vi "custom_2_stimulus_setup.vi"(1 "input cluster":T1) -> (0 "output cluster":T2)   [LabVIEW 2010]
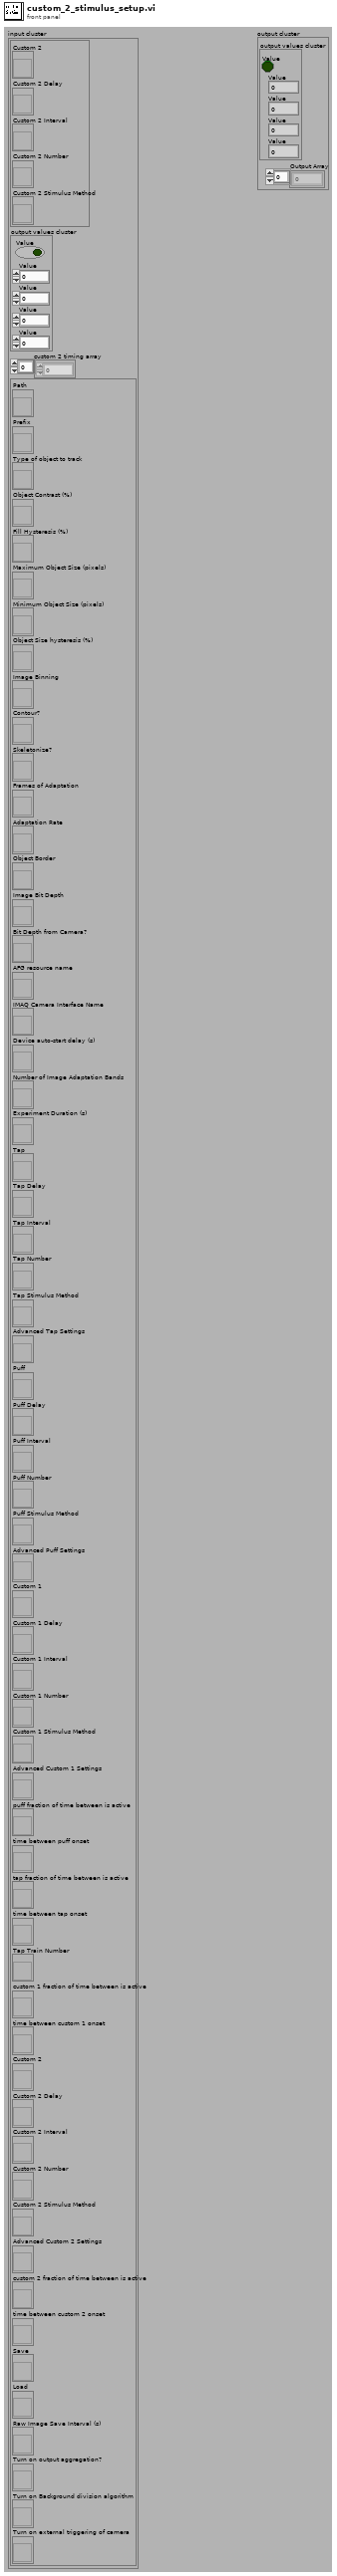
[diagram p1: front panel]
types:
  T1 = cluster{cluster{"Custom 2":refnum<vi>, "Custom 2 Delay":refnum<vi>, "Custom 2 Interval":refnum<vi>, "Custom 2 Number":refnum<vi>, "Custom 2 Stimulus Method":refnum<vi>}, "output values cluster":cluster{"Value":bool, "Value":dbl, "Value":dbl, "Value":dbl, "Value":u16}, "custom 2 timing array":dbl[], cluster{"Path":refnum<vi>, "Prefix":refnum<vi>, "Type of object to track":refnum<vi>, "Object Contrast (%)":refnum<vi>, "Fill Hysteresis (%)":refnum<vi>, "Maximum Object Size (pixels)":refnum<vi>, "Minimum Object Size (pixels)":refnum<vi>, "Object Size hysteresis (%)":refnum<vi>, "Image Binning":refnum<vi>, "Contour?":refnum<vi>, "Skeletonize?":refnum<vi>, "Frames of Adaptation":refnum<vi>, "Adaptation Rate":refnum<vi>, "Object Border":refnum<vi>, "Image Bit Depth":refnum<vi>, "Bit Depth from Camera?":refnum<vi>, "AFG resource name":refnum<vi>, "IMAQ Camera Interface Name":refnum<vi>, "Device auto-start delay (s)":refnum<vi>, "Number of Image Adaptation Bands":refnum<vi>, "Experiment Duration (s)":refnum<vi>, "Tap":refnum<vi>, "Tap Delay":refnum<vi>, "Tap Interval":refnum<vi>, "Tap Number":refnum<vi>, "Tap Stimulus Method":refnum<vi>, "Advanced Tap Settings":refnum<vi>, "Puff":refnum<vi>, "Puff Delay":refnum<vi>, "Puff Interval":refnum<vi>, "Puff Number":refnum<vi>, "Puff Stimulus Method":refnum<vi>, "Advanced Puff Settings":refnum<vi>, "Custom 1":refnum<vi>, "Custom 1 Delay":refnum<vi>, "Custom 1 Interval":refnum<vi>, "Custom 1 Number":refnum<vi>, "Custom 1 Stimulus Method":refnum<vi>, "Advanced Custom 1 Settings":refnum<vi>, "puff fraction of time between is active":refnum<vi>, "time between puff onset":refnum<vi>, "tap fraction of time between is active":refnum<vi>, "time between tap onset":refnum<vi>, "Tap Train Number":refnum<vi>, "custom 1 fraction of time between is active":refnum<vi>, "time between custom 1 onset":refnum<vi>, "Custom 2":refnum<vi>, "Custom 2 Delay":refnum<vi>, "Custom 2 Interval":refnum<vi>, "Custom 2 Number":refnum<vi>, "Custom 2 Stimulus Method":refnum<vi>, "Advanced Custom 2 Settings":refnum<vi>, "custom 2 fraction of time between is active":refnum<vi>, "time between custom 2 onset":refnum<vi>, "Save":refnum<vi>, "Load":refnum<vi>, "Raw Image Save Interval (s)":refnum<vi>, "Turn on output aggregation?":refnum<vi>, "Turn on Background division algorithm":refnum<vi>, "Turn on external triggering of camera":refnum<vi>}}
  T2 = cluster{"output values cluster":cluster{"Value":bool, "Value":dbl, "Value":dbl, "Value":dbl, "Value":u16}, "Output Array":dbl[]}
  T3 = cluster{"Custom 2":refnum<vi>, "Custom 2 Delay":refnum<vi>, "Custom 2 Interval":refnum<vi>, "Custom 2 Number":refnum<vi>, "Custom 2 Stimulus Method":refnum<vi>}
  T4 = cluster{"Value":bool, "Value":dbl, "Value":dbl, "Value":dbl, "Value":u16}
  T5 = cluster{"Path":refnum<vi>, "Prefix":refnum<vi>, "Type of object to track":refnum<vi>, "Object Contrast (%)":refnum<vi>, "Fill Hysteresis (%)":refnum<vi>, "Maximum Object Size (pixels)":refnum<vi>, "Minimum Object Size (pixels)":refnum<vi>, "Object Size hysteresis (%)":refnum<vi>, "Image Binning":refnum<vi>, "Contour?":refnum<vi>, "Skeletonize?":refnum<vi>, "Frames of Adaptation":refnum<vi>, "Adaptation Rate":refnum<vi>, "Object Border":refnum<vi>, "Image Bit Depth":refnum<vi>, "Bit Depth from Camera?":refnum<vi>, "AFG resource name":refnum<vi>, "IMAQ Camera Interface Name":refnum<vi>, "Device auto-start delay (s)":refnum<vi>, "Number of Image Adaptation Bands":refnum<vi>, "Experiment Duration (s)":refnum<vi>, "Tap":refnum<vi>, "Tap Delay":refnum<vi>, "Tap Interval":refnum<vi>, "Tap Number":refnum<vi>, "Tap Stimulus Method":refnum<vi>, "Advanced Tap Settings":refnum<vi>, "Puff":refnum<vi>, "Puff Delay":refnum<vi>, "Puff Interval":refnum<vi>, "Puff Number":refnum<vi>, "Puff Stimulus Method":refnum<vi>, "Advanced Puff Settings":refnum<vi>, "Custom 1":refnum<vi>, "Custom 1 Delay":refnum<vi>, "Custom 1 Interval":refnum<vi>, "Custom 1 Number":refnum<vi>, "Custom 1 Stimulus Method":refnum<vi>, "Advanced Custom 1 Settings":refnum<vi>, "puff fraction of time between is active":refnum<vi>, "time between puff onset":refnum<vi>, "tap fraction of time between is active":refnum<vi>, "time between tap onset":refnum<vi>, "Tap Train Number":refnum<vi>, "custom 1 fraction of time between is active":refnum<vi>, "time between custom 1 onset":refnum<vi>, "Custom 2":refnum<vi>, "Custom 2 Delay":refnum<vi>, "Custom 2 Interval":refnum<vi>, "Custom 2 Number":refnum<vi>, "Custom 2 Stimulus Method":refnum<vi>, "Advanced Custom 2 Settings":refnum<vi>, "custom 2 fraction of time between is active":refnum<vi>, "time between custom 2 onset":refnum<vi>, "Save":refnum<vi>, "Load":refnum<vi>, "Raw Image Save Interval (s)":refnum<vi>, "Turn on output aggregation?":refnum<vi>, "Turn on Background division algorithm":refnum<vi>, "Turn on external triggering of camera":refnum<vi>}
  T6 = cluster{"custom 2 fraction of time between is active":refnum<vi>, "time between custom 2 onset":refnum<vi>}
  T7 = cluster{"Custom":refnum<vi>, "Custom Delay":refnum<vi>, "Custom Interval":refnum<vi>, "Custom Number":refnum<vi>, "Custom Stimulus Method":refnum<vi>}
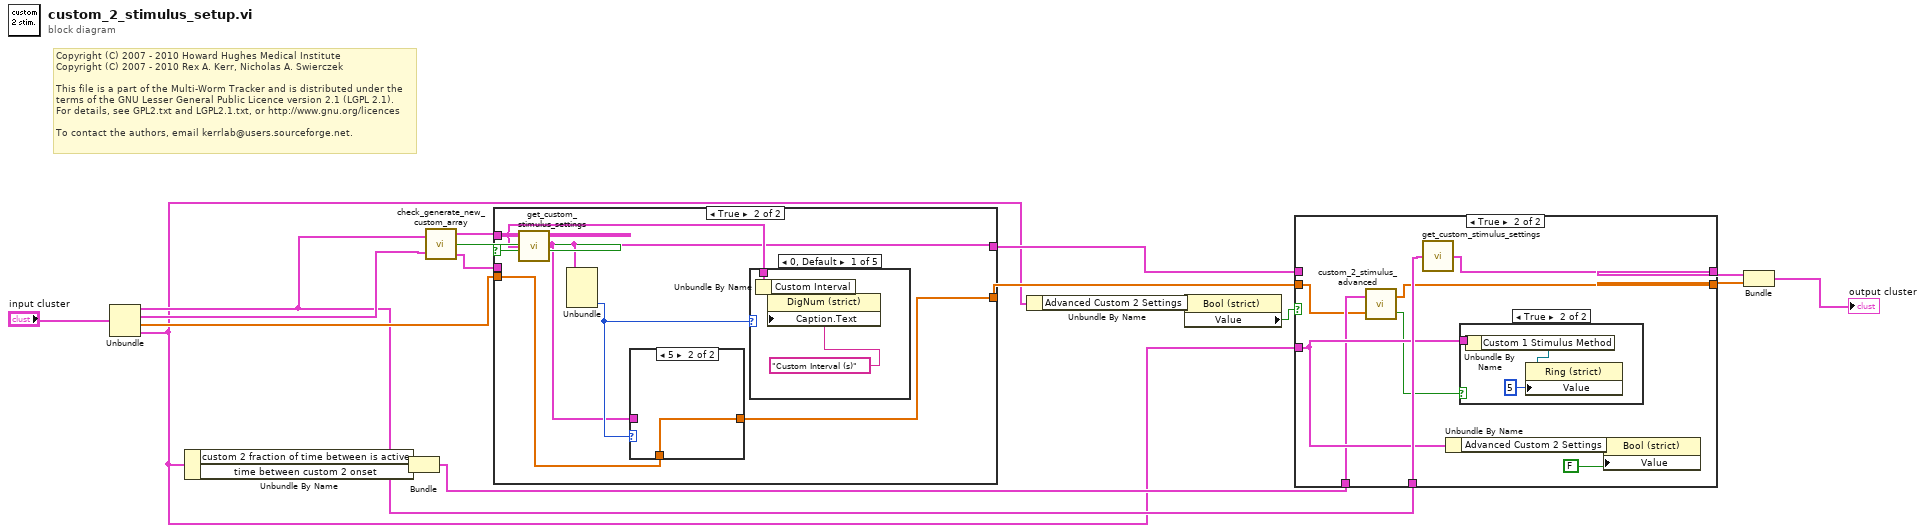
[diagram p0: block diagram]
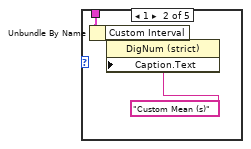
[diagram p5: hidden frame]
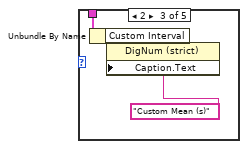
[diagram p6: hidden frame]
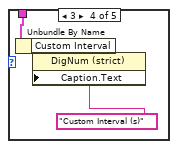
[diagram p7: hidden frame]
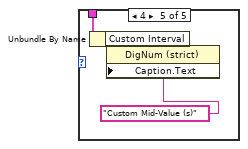
[diagram p8: hidden frame]
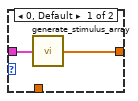
[diagram p9: hidden frame]
diagram:
  # "Copyright (C) 2007 - 2010 Howard Hughes Medical Institute\nCopyright (C) 2007 - 2010 Rex A. Kerr, Nicholas A. Swierczek\n \nThis file is a part of the Multi-Worm Tracker and is distributed under the\nterms of the GNU Lesser General Public Licence version 2.1 (LGPL 2.1).\nFor details, see GPL2.txt and LGPL2.1.txt, or http://www.gnu.org/licences\n \nTo contact the authors, email kerrlab@users.sourceforge.net."
  n1 = Unbundle("input cluster") -> (w6:T3, "output values cluster"=w7:T4, "custom 2 timing array"=w16:dbl[], w4:T5)
  n2 = Unbundle By Name(w4) -> ("custom 2 fraction of time between is active"=w15:refnum<vi>, "time between custom 2 onset"=w14:refnum<vi>)
  n3 = Bundle("custom 2 fraction of time between is active"=w15, "time between custom 2 onset"=w14) -> (w13:T6)  [unwired: 1 in]
  n4 = call "check_generate_new_custom_array.vi"("Cluster"=w6, "output values cluster"=w7) -> ("output cluster"=w10:T7, "Need new custom array?"=w9:bool, "Output values cluster"=w8:T4)
  n5 = case shown="True" w9 {
    tunnel: w10 -> [_ w22]
    tunnel: w8 -> [w20 _]
    tunnel: [w20 w21] -> w17
    tunnel: [w19 w25] -> w18
    tunnel: w16 -> [w19 w24]
    frame False {
    }
    frame True {
      n6 = call "get_custom_stimulus_settings.vi"("input references cluster"=w22) -> ("output values cluster"=w21:T4)
      n7 = Unbundle(w21) -> ("Value"=w23:u16)  [unwired: 4 out]
      n8 = case shown="5" w23 {
        tunnel: [w42 w43] -> w25
        tunnel: w21 -> [w41 _]
        tunnel: w24 -> [_ w43]
        frame 0, Default {
          n9 = call "generate_stimulus_array.vi"("Values Cluster"=w41) -> ("Array"=w42:dbl[])
        }
        frame 5 {
        }
      }
      n10 = case shown="0, Default" w23 {
        tunnel: w22 -> [w28 w30 w32 w35 w38]
        frame 0, Default {
          n11 = Unbundle By Name(w28) -> ("Custom Interval"=w27:refnum<vi>)
          n12 = property class="DigNum (strict)"(reference=w27, "Caption.Text"="Custom Interval (s)") -> ()  [unwired: 1 in, 2 out]
        }
        frame 1 {
          n13 = Unbundle By Name(w30) -> ("Custom Interval"=w31:refnum<vi>)
          n14 = property class="DigNum (strict)"(reference=w31, "Caption.Text"="Custom Mean (s)") -> ()  [unwired: 1 in, 2 out]
        }
        frame 2 {
          n15 = Unbundle By Name(w32) -> ("Custom Interval"=w34:refnum<vi>)
          n16 = property class="DigNum (strict)"(reference=w34, "Caption.Text"="Custom Mean (s)") -> ()  [unwired: 1 in, 2 out]
        }
        frame 3 {
          n17 = Unbundle By Name(w35) -> ("Custom Interval"=w37:refnum<vi>)
          n18 = property class="DigNum (strict)"(reference=w37, "Caption.Text"="Custom Interval (s)") -> ()  [unwired: 1 in, 2 out]
        }
        frame 4 {
          n19 = Unbundle By Name(w38) -> ("Custom Interval"=w40:refnum<vi>)
          n20 = property class="DigNum (strict)"(reference=w40, "Caption.Text"="Custom Mid-Value (s)") -> ()  [unwired: 1 in, 2 out]
        }
      }
    }
  }
  n21 = Unbundle By Name(w4) -> ("Advanced Custom 2 Settings"=w5:refnum<vi>)
  n22 = property class="Bool (strict)"(reference=w5) -> ("Value"=w3:bool)  [unwired: 1 in, 2 out]
  n23 = case shown="True" w3 {
    tunnel: w18 -> [w45 w48]
    tunnel: [w45 w47] -> w11
    tunnel: w4 -> [_ w50]
    tunnel: w13 -> [_ w49]
    tunnel: w17 -> [w44 _]
    tunnel: [w44 w53] -> w12
    tunnel: w6 -> [_ w54]
    frame False {
    }
    frame True {
      n24 = call "custom_2_stimulus_advanced.vi"("Input Array"=w48, "Cluster"=w49) -> ("Timing array changed?"=w46:bool, "Output Array"=w47:dbl[])
      n25 = call "get_custom_stimulus_settings.vi"("input references cluster"=w54) -> ("output values cluster"=w53:T4)
      n26 = Unbundle By Name(w50) -> ("Advanced Custom 2 Settings"=w51:refnum<vi>)
      n27 = case shown="True" w46 {
        tunnel: w50 -> [_ w55]
        frame False {
        }
        frame True {
          n28 = Unbundle By Name(w55) -> ("Custom 1 Stimulus Method"=w56:refnum<vi>)
          n29 = property class="Ring (strict)"(reference=w56, "Value"=u16 5) -> ()  [unwired: 1 in, 2 out]
        }
      }
      n30 = property class="Bool (strict)"(reference=w51, "Value"=FALSE) -> ()  [unwired: 1 in, 2 out]
    }
  }
  n31 = Bundle("output values cluster"=w12, "Output Array"=w11) -> (→"output cluster":T2)  [unwired: 1 in]
